vi "Random Number Range.vi"() -> ()   [LabVIEW 2020]
uses:
  <vilib>/numeric/Random Number (Range) U64.vi
  <vilib>/numeric/sub_Random U32.vi
panel:
  out "number":u64
  in  "lower bound (0)":u64
  in  "upper bound (100)":u64=100
  # "Random Number Range"
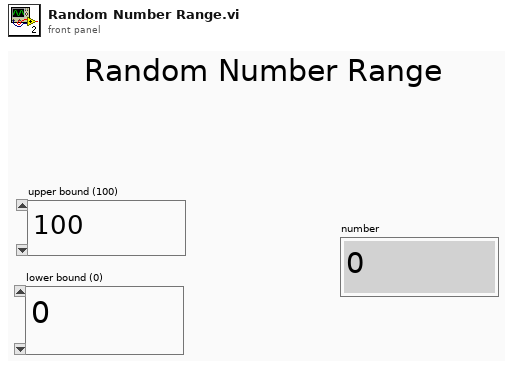
[diagram p1: front panel]
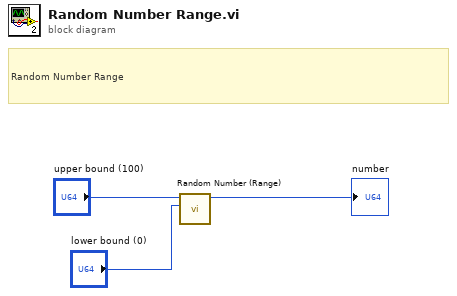
[diagram p0: block diagram]
diagram:
  # "Random Number Range"
  n1 = call-poly <vilib>:"Random Number (Range).vi"("lower bound (0)"="lower bound (0)", "upper bound (100)"="upper bound (100)") -> ("number"=→"number":u64)  [unwired: 9 in]
